vi "DM pop burst.vi"(8 "error in (no error)":errorcluster, 11 "group":string) -> (0 "error out":errorcluster, 3 "burst":refnum<class "mmWave data.lvclass">)   [LabVIEW 2019, in "DataManagment.lvlib"]
uses:
  DataManagment.lvlib
  SubVIs/mmWave data_class/mmWave data.lvclass
  DM get burst parameters.ctl
  <vilib>/Utility/error.llb/Error Cluster From Error Code.vi
  <vilib>/ErrorRing/Error Ring.xnode
  <vilib>/addons/_JKI.lib/Serialization/JSON/JKI JSON Serialization.lvlib
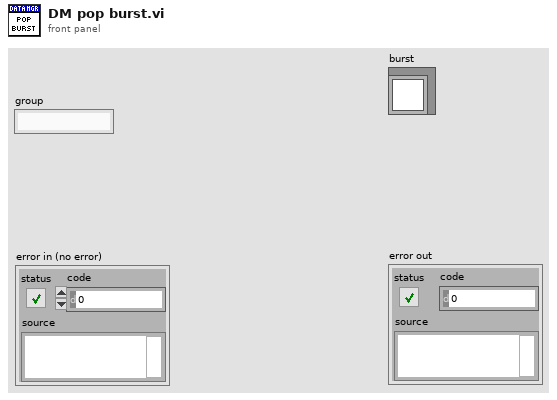
[diagram p1: front panel]
types:
  T1 = typedef "DataManagment.lvlib/DM get burst parameters.ctl" = cluster{"group":string, "bursts":string[]}
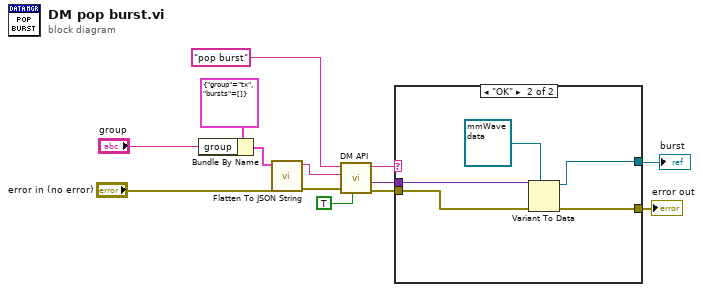
[diagram p0: block diagram]
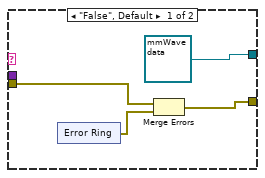
[diagram p2: hidden frame]
diagram:
  n1 = Bundle By Name(cluster=T1 {"group"="tx", "bursts"=[]} ("Cluster"), "group"="group") -> (w5:T1)
  n2 = call <vilib>:"Flatten To JSON String.vi"("error in (no error)"="error in (no error)", "Variant"=w5) -> ("error out"=w3:errorcluster, "JSON String"=w2:string)  [unwired: 8 in]
  n3 = call "DM API.vi"("response"=TRUE, "error in (no error)"=w3, "parameters"=w2, "message"="pop burst") -> ("error out"=w8:errorcluster, "data"=w10:variant, "status"=w11:string)  [unwired: 4 in, 1 out]
  n4 = case shown="\"OK\"" w11 {
    tunnel: w10 -> [_ w27]
    tunnel: [refnum<class "mmWave data.lvclass"> refnum ("mmWave data") w23] -> w9
    tunnel: [w15 w24] -> w7
    tunnel: w8 -> [w14 w25]
    frame "False", Default {
      n5 = xnode "Error Ring"() -> ("error out"=w16:errorcluster)
      n6 = Merge Errors(w14, w16) -> (w15:errorcluster)
    }
    frame "OK" {
      n7 = Variant To Data(error in=w25, type=refnum<class "mmWave data.lvclass"> refnum ("Array"), Variant=w27) -> (data=w23:refnum<class "mmWave data.lvclass">, error out=w24:errorcluster)
    }
  }
  "burst" <- w9
  "error out" <- w7
